vi "Untitled 1.vi"() -> ()   [LabVIEW 2020]
uses:
  FPGA/Libraries/Raster/Triangle.ctl
  FPGA/Libraries/Raster/Vertex.ctl
  FPGA/Libraries/Raster/Vector 3D.ctl
  FPGA/Libraries/Raster/UV.ctl
  <vilib>/rvi/interface/common/niFpgaWaitOnOcc.vi
  <vilib>/Utility/error.llb/Error Cluster From Error Code.vi
  <vilib>/rvi/errors/niLvFpgaAdjustHostInterfaceError.vi
  <vilib>/rvi/interface/nirviOpenFPGA/nirviOpenFPGA.xnode
  Builds/FPGA/TestDRAM.lvbitx
  FPGA/Libraries/Raster/Test - With DRAM.vi
  <vilib>/rvi/interface/nirviMethod/nirviMethod.xnode
  <vilib>/rvi/interface/nirviReadWriteControl/nirviReadWriteControl.xnode
  <vilib>/rvi/errors/niLvFpgaMergeErrorWithErrorCode.vi
  <vilib>/FPGAPlugInAG/PXI-7952R/niLvFpga_ReadFifo_PXI-7952R.vi
  NiFpgaLv.dll
  FPGA/Libraries/Raster/Raster (FPGA).lvlib
  <vilib>/FPGAPlugInAG/PXI-7952R/niLvFpga_Open_PXI-7952R.vi
  <vilib>/FPGAPlugInAG/PXI-7952R/niLvFpga_ConfigureFifo_PXI-7952R.vi
  <vilib>/FPGAPlugInAG/PXI-7952R/niLvFpga_StartFifo_PXI-7952R.vi
  <vilib>/FPGAPlugInAG/PXI-7952R/niLvFpga_Reset_PXI-7952R.vi
  <vilib>/FPGAPlugInAG/PXI-7952R/niLvFpga_Run_PXI-7952R.vi
panel:
  in  "Send To Host":bool
  out "Latest Data":cluster{"Address":i32, "Value":u32}
  out "Numeric":u32
  out "Waveform Graph":u32[](graph)
  out "Data 2":u32[](array[numeric]) format="%.0x"
  out "Actual Depth":u32
  out "DRAM Read Address":u32
  out "To DRAM Timed Out?":bool
  out "Raster Loop Index":i32
  out "Data":u32[](array[numeric])
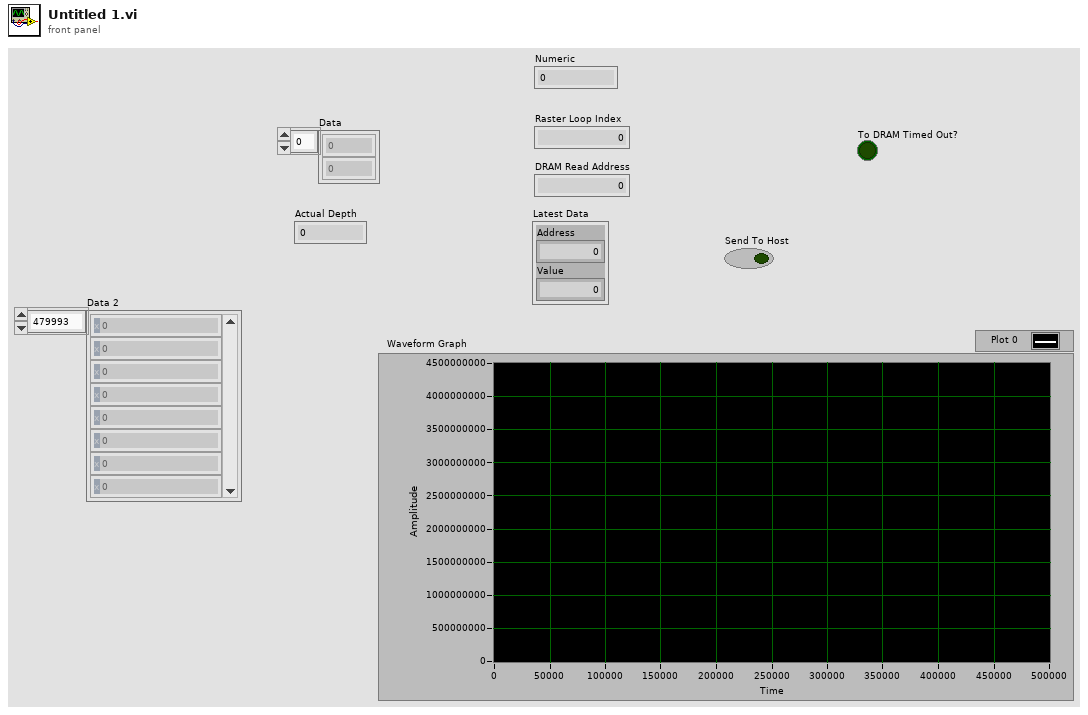
[diagram p1: front panel]
types:
  T1 = typedef "Raster (FPGA).lvlib/Triangle.ctl" = cluster{"Vertex 1":T2, "Vertex 2":T2, "Vertex 3":T2, "Colour":u32}
  T2 = typedef "Raster (FPGA).lvlib/Vertex.ctl" = cluster{"Position":T3, "UV":T4, "Colour":u32}
  T3 = typedef "Raster (FPGA).lvlib/Vector 3D.ctl" = cluster{"x":sgl, "y":sgl, "z":sgl}
  T4 = typedef "Raster (FPGA).lvlib/UV.ctl" = cluster{"u":sgl, "v":sgl}
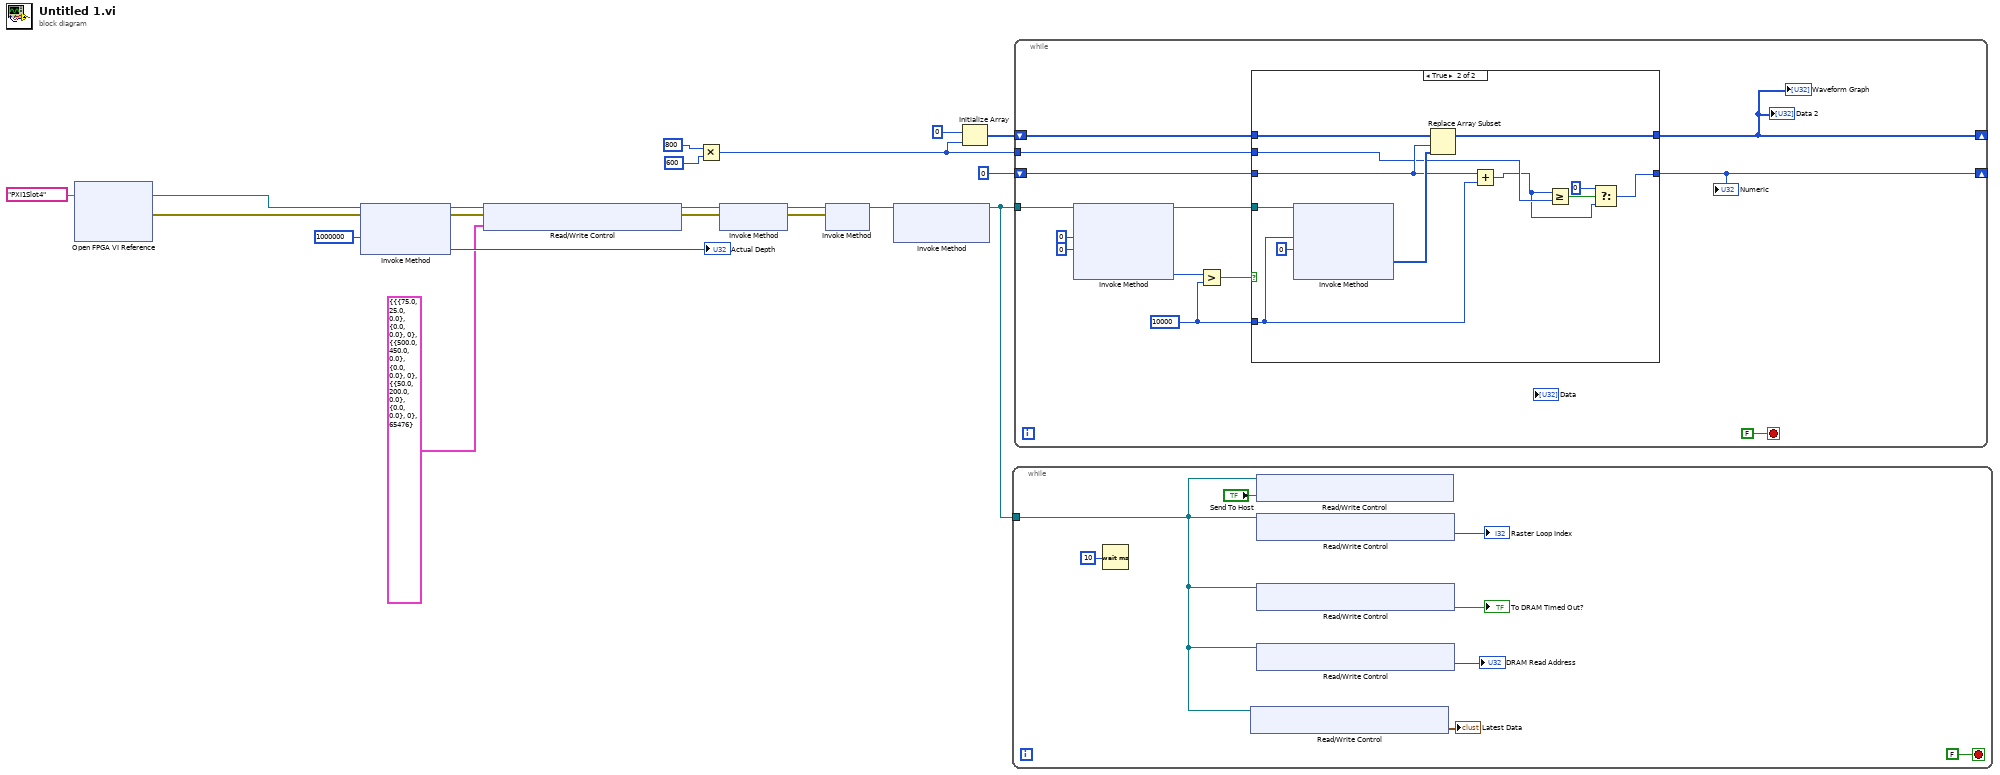
[diagram p0: block diagram]
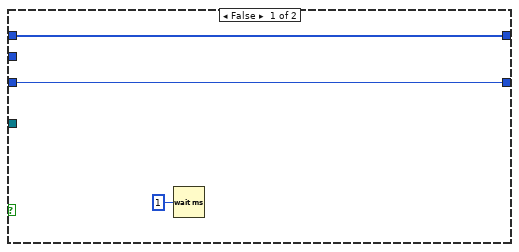
[diagram p2: hidden frame]
diagram:
  n1 = xnode "Open FPGA VI Reference"("resource name"=tag "PXI1Slot4") -> ("FPGA VI Reference Out"=w16:refnum<k20>, "error out"=w15:errorcluster)  [unwired: 1 in]
  n2 = xnode "Invoke Method"("FPGA VI Reference In"=w16, "error in"=w15, "Requested Depth"=u32 1000000) -> ("FPGA VI Reference Out"=w6:refnum<k20>, "error out"=w5:errorcluster, "Actual Depth"=→"Actual Depth":u32)
  n3 = xnode "Read/Write Control"("FPGA VI Reference In"=w6, "error in"=w5, "Triangle"=T1 {"Vertex 1"={"Position"={"x"=75.0, "y"=25.0, "z"=0.0}, "UV"={"u"=0.0, "v"=0.0}, "Colour"=0}, "Vertex 2"={"Position"={"x"=500.0, "y"=450.0, "z"=0.0}, "UV"={"u"=0.0, "v"=0.0}, "Colour"=0}, "Vertex 3"={"Position"={"x"=50.0, "y"=200.0, "z"=0.0}, "UV"={"u"=0.0, "v"=0.0}, "Colour"=0}, "Colour"=65476}) -> ("FPGA VI Reference Out"=w4:refnum<k20>, "error out"=w3:errorcluster)
  n4 = Multiply(x=u32 800, y=u32 600) -> (x*y=w1:u32)
  n5 = xnode "Invoke Method"("FPGA VI Reference In"=w4, "error in"=w3) -> ("FPGA VI Reference Out"=w19:refnum<k20>, "error out"=w18:errorcluster)
  n6 = xnode "Invoke Method"("FPGA VI Reference In"=w19, "error in"=w18) -> ("FPGA VI Reference Out"=w17:refnum<k20>)  [unwired: 1 out]
  n7 = xnode "Invoke Method"("FPGA VI Reference In"=w17) -> ("FPGA VI Reference Out"=w12:refnum<k20>)  [unwired: 2 in, 1 out]
  n8 = Initialize Array(u32 0, w1) -> (w11:u32[])
  n9 = while {
    tunnel: w12 -> [w22]
    stop <- FALSE stop-if-true
    n10 = Wait (ms)(milliseconds to wait=u32 10) -> ()  [unwired: 1 out]
    n11 = xnode "Read/Write Control"("FPGA VI Reference In"=w22) -> ("Latest Data"=→"Latest Data":cluster{"Address":i32, "Value":u32})  [unwired: 1 in, 2 out]
    n12 = xnode "Read/Write Control"("FPGA VI Reference In"=w22, "Send To Host"="Send To Host") -> ()  [unwired: 1 in, 2 out]
    n13 = xnode "Read/Write Control"("FPGA VI Reference In"=w22) -> ("Raster Loop Index"=→"Raster Loop Index":i32)  [unwired: 1 in, 2 out]
    n14 = xnode "Read/Write Control"("FPGA VI Reference In"=w22) -> ("To DRAM Timed Out?"=→"To DRAM Timed Out?":bool)  [unwired: 1 in, 2 out]
    n15 = xnode "Read/Write Control"("FPGA VI Reference In"=w22) -> ("DRAM Read Address"=→"DRAM Read Address":u32)  [unwired: 1 in, 2 out]
  }
  n16 = while {
    tunnel: w12 -> [w41]
    shift-right: [w31] -> _
    shift-left: w11 -> [w34]
    shift-right: [w32] -> _
    shift-left: 0 -> [w33]
    tunnel: w1 -> [w29]
    stop <- FALSE stop-if-true
    w36 = u32 10000 ("y")
    n17 = xnode "Invoke Method"("FPGA VI Reference In"=w41, "Number of Elements"=u32 0, "Timeout (ms)"=0) -> ("FPGA VI Reference Out"=w35:refnum<k20>, "Elements Remaining"=w38:u32)  [unwired: 1 in, 2 out]
    n18 = Greater?(x=w38, y=w36) -> (0:w37:bool)
    n19 = case shown="True" w37 {
      tunnel: w36 -> [_ w51]
      tunnel: w35 -> [_ w55]
      tunnel: w34 -> [w44 w54]
      tunnel: [w44 w52] -> w31
      tunnel: w33 -> [w43 w50]
      tunnel: [w43 w45] -> w32
      tunnel: w29 -> [_ w49]
      frame False {
        n20 = Wait (ms)(milliseconds to wait=u32 1) -> ()  [unwired: 1 out]
      }
      frame True {
        n21 = xnode "Invoke Method"("FPGA VI Reference In"=w55, "Number of Elements"=w51, "Timeout (ms)"=0) -> ("Data"=w53:u32[])  [unwired: 1 in, 3 out]
        n22 = Replace Array Subset(array=w54, new element=w53, index=w50) -> (w52:u32[])
        n23 = Add(x=w50, y=w51) -> (x+y=w46:u32)
        n24 = Greater Or Equal?(x=w46, y=w49) -> (x >= y?=w48:bool)
        n25 = Select(t=u32 0, s=w48, f=w46) -> (s? t:f=w45:u32)
      }
    }
    "Data 2" <- w31
    "Waveform Graph" <- w31
    "Numeric" <- w32
  }
